vi "solar_write SOLARUIPanes.vi"(8 "error in (no error)":errorcluster, 10 "Panes":T1={"Status"=TRUE, "Emergency"=TRUE, "Targets"=TRUE}, 11 "solar in":refnum<class "solar.lvclass">) -> (0 "error out":errorcluster, 3 "solar out":refnum<class "solar.lvclass">)   [LabVIEW 2018, in "solar.lvclass"]
doc: "This shows/hides the different window panes in the SOLAR user interface. If Targets pane is hidden, the Emergency pane is always hidden."
uses:
  solar.lvclass
  solar_ctl SOLAR UI Panes.ctl
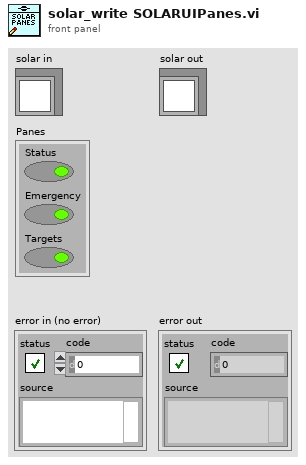
[diagram p1: front panel]
types:
  T1 = typedef "solar_ctl SOLAR UI Panes.ctl" = cluster{"Status":bool, "Emergency":bool, "Targets":bool}
  T2 = typedef "solar_ctl SOLAR Refnum.ctl" = refnum<k1>
  T3 = typedef "solar_ctl SOLAR Global.ctl" = cluster{"Targets":T4[], "AppDir":path, "solar.ini":path, "ConfigsDir":path, "CosmosDir":path, "LogsDir":path, "ExePath":path, "ExeVersion":string, "PartNum":string, "AppSetup":string, "Title":string, "Main.ini":path, "Temp.ini":path, "vSOLAR":string, "Splash.png":string, "SplashWait":i32, "SOLARUE":refnum<user-event>, "VoyagerRefnum":T5, "QTimerRefnum":T6}
  T4 = typedef "solar_ctl Target Global.ctl" = cluster{"Target":string, "Q":refnum<queue>, "UE":refnum<user-event>, "VI":refnum<vi>, "Menu":refnum<k9>, "Data":refnum<data-value>, "Attributes":variant}
  T5 = typedef "solar_voy_ctl Voyager Refnum.ctl" = refnum<k1>
  T6 = typedef "solar_qtimer_ctl Refnum.ctl" = refnum<k1>
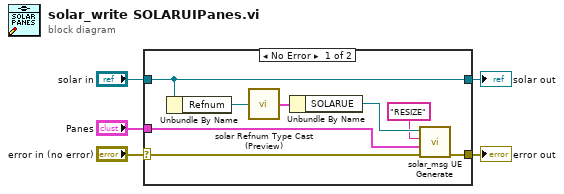
[diagram p0: block diagram]
diagram:
  n1 = case shown="No Error" "error in (no error)" {
    selector: "error in (no error)" -> [w12 w15]
    tunnel: [w13 w15] -> w5
    tunnel: "Panes" -> [w6 _]
    tunnel: "solar in" -> [w8 w14]
    tunnel: [w8 w14] -> w1
    frame No Error {
      n2 = Unbundle By Name(w8) -> ("Refnum"=w11:T2)
      n3 = call "solar Refnum Type Cast (Preview).vi"("Refnum"=w11) -> ("SOLAR"=w10:T3)  [unwired: 8 in]
      n4 = Unbundle By Name(w10) -> ("SOLARUE"=w9:refnum<user-event>)
      n5 = call "solar_msg UE Generate.vi"("error in (no error)"=w12, "CMD_DATA (Last)"=w6, "CMD (Last)"="RESIZE" ("Packet"), "UserEvent in"=w9) -> ("error out"=w13:errorcluster)  [unwired: 6 in, 1 out]
    }
    frame Error {
    }
  }
  "error out" <- w5
  "solar out" <- w1
